vi "changeState.vi"(8 "error in (no error)":errorcluster, 10 "StateValue":T1, 11 "ElectrometerController in":refnum<class "ElectrometerController.lvclass">) -> (0 "error out":errorcluster, 3 "ElectrometerController out":refnum<class "ElectrometerController.lvclass">)   [LabVIEW 2016, in "ElectrometerController.lvclass"]
uses:
  ElectrometerController.lvclass
  ts_electrometeruserevents/Typedefs/StateValue.ctl
  Electrometer/State/ReadyState.lvclass
  home/andres/ts_electrometer/ss_electrometer/Electrometer/State/ElectrometerState.lvclass
  Electrometer/State/ConfiguringState.lvclass
  Electrometer/State/ManualReadingState.lvclass
  Electrometer/State/UntilIntensityReadingState/UntilIntensityReading.lvclass
  Electrometer/State/SetDurationReadingState/SetDurationReading.lvclass
  Electrometer/State/ReadingBufferState/ReadingBufferState.lvclass
  Electrometer/State/StandByState/ElectrometerStandByState.lvclass
  Electrometer/State/DisabledState/ElectrometerDisabledState.lvclass
  ts_electrometeruserevents/Typedefs/ElectrometerTypedefs.lvlib
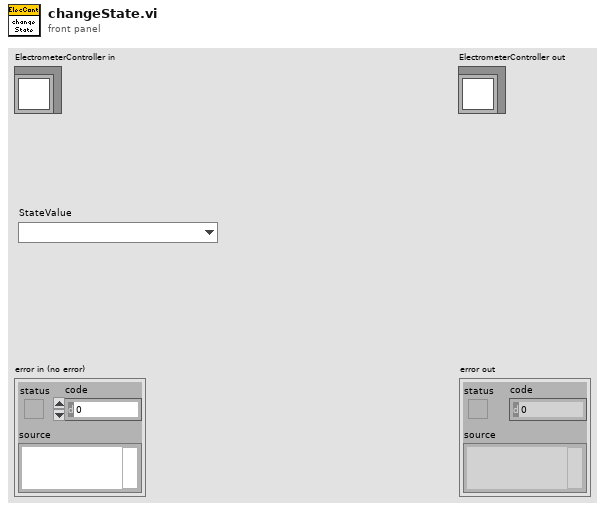
[diagram p1: front panel]
types:
  T1 = typedef "ElectrometerTypedefs.lvlib/StateValue.ctl" = enum16{"", "DisabledState", "EnabledState", "FaultState", "OffState", "StandbyState", "ReadyState", "ConfiguringState", "ManualReadingState", "UntilIntensityReadingState", "SetDurationReadingState", "BufferReadingState"}
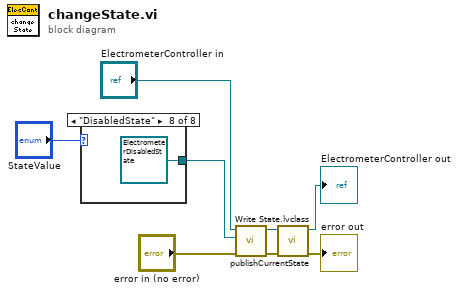
[diagram p0: block diagram]
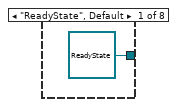
[diagram p2: hidden frame]
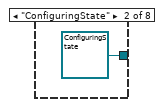
[diagram p3: hidden frame]
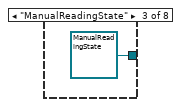
[diagram p4: hidden frame]
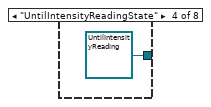
[diagram p5: hidden frame]
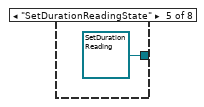
[diagram p6: hidden frame]
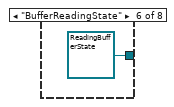
[diagram p7: hidden frame]
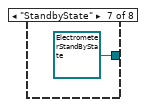
[diagram p8: hidden frame]
diagram:
  n1 = case shown="\"DisabledState\"" "StateValue" {
    tunnel: [refnum<class "ReadyState.lvclass"> refnum ("ReadyState.lvclass") refnum<class "ConfiguringState.lvclass"> refnum ("ConfiguringState.lvclass") refnum<class "ManualReadingState.lvclass"> refnum ("ManualReadingState.lvclass") refnum<class "UntilIntensityReading.lvclass"> refnum ("UntilIntensityReading.lvclass") refnum<class "SetDurationReading.lvclass"> refnum ("SetDurationReading.lvclass") refnum<class "ReadingBufferState.lvclass"> refnum ("ReadingBufferState.lvclass") refnum<class "ElectrometerStandByState.lvclass"> refnum ("ElectrometerStandByState.lvclass") refnum<class "ElectrometerDisabledState.lvclass"> refnum ("ElectrometerDisabledState.lvclass")] -> w7
    frame "ReadyState", Default {
    }
    frame "ConfiguringState" {
    }
    frame "ManualReadingState" {
    }
    frame "UntilIntensityReadingState" {
    }
    frame "SetDurationReadingState" {
    }
    frame "BufferReadingState" {
    }
    frame "StandbyState" {
    }
    frame "DisabledState" {
    }
  }
  n2 = call-dynamic "Write State.lvclass.vi"("error in (no error)"="error in (no error)", "ElectrometerState"=w7, "ElectrometerController in"="ElectrometerController in") -> ("error out"=w3:errorcluster, "ElectrometerController out"=w5:refnum<class "ElectrometerController.lvclass">)  [unwired: 7 in]
  n3 = call "publishCurrentState.vi"("error in (no error)"=w3, "ElectrometerController in"=w5) -> ("error out"=→"error out":errorcluster, "ElectrometerController out"=→"ElectrometerController out":refnum<class "ElectrometerController.lvclass">)  [unwired: 8 in]
